vi "Write Data.vi"(8 "error in (no error)":errorcluster, 9 "Publication Time":timestamp, 10 "Value":variant, 11 "FormattedStringBinding In":refnum<class "FormattedStringBinding.lvclass">) -> (0 "error out":errorcluster, 3 "FormattedStringBinding Out":refnum<class "FormattedStringBinding.lvclass">)   [LabVIEW 2019, in "FormattedStringBinding.lvclass"]
doc: "<License>\nCopyright © 2017 Composed Systems, LLC | All rights reserved\nwww.composed.io\n\nAuthor: Ethan Stern <ethan.stern@composed.io>\n\nThis software is provided \"AS IS\" WITHOUT WARRANTIES, either express or implied, AND IS FOR EDUCATIONAL PURPOSES ONLY.\n</License>"
uses:
  <vilib>/gpm_packages/@cs/transport/Source/Concrete/FormattedStringBinding/FormattedStringBinding.lvclass
  <vilib>/gpm_packages/@cs/transport/Source/Concrete/FormattedStringBinding/FormattedStringBinding.lvclass/FormattedStringBinding.ctl
  <vilib>/Utility/error.llb/Error Cluster From Error Code.vi
  <vilib>/gpm_packages/@cs/transport/Source/Concrete/TerminalValueBinding/TerminalValueBinding.lvclass
  <vilib>/ErrorRing/Error Ring.xnode
  <vilib>/Utility/Data Type/NI_Data Type.lvlib
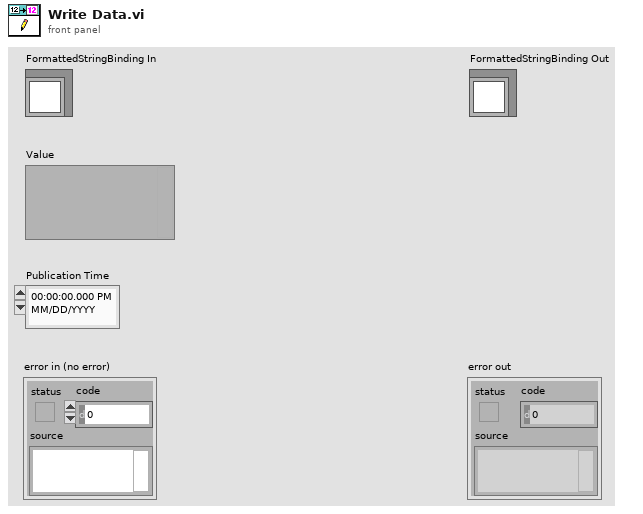
[diagram p1: front panel]
types:
  T1 = typedef "NI_Data Type.lvlib/Data Type.ctl" = enum8{"Invalid Type", "Void", "I8", "I16", "I32", "I64", "U8", "U16", "U32", "U64", "Single Float", "Double Float", "Extended Float", "Single Complex", "Double Complex", "Extended Complex", "Enum U8", "Enum U16", "Enum U32", "Enum U64", "Single Float With Unit", "Double Float With Unit", "Extended Float With Unit", "Single Complex with Unit", "Double Complex with Unit", "Extended Complex with Unit", "Boolean", "String", "Path", "Picture", "Tag", "Array", "Cluster", "Variant", "LV Variant", "Waveform", "Timestamp", "Digital Waveform", "Digital Data", "ExpressData", "Refnum", "External Data", "VI", "Poly VI", "LabVIEW Class Instance", "Fixed Point", "Set Collection", "Map Collection"}
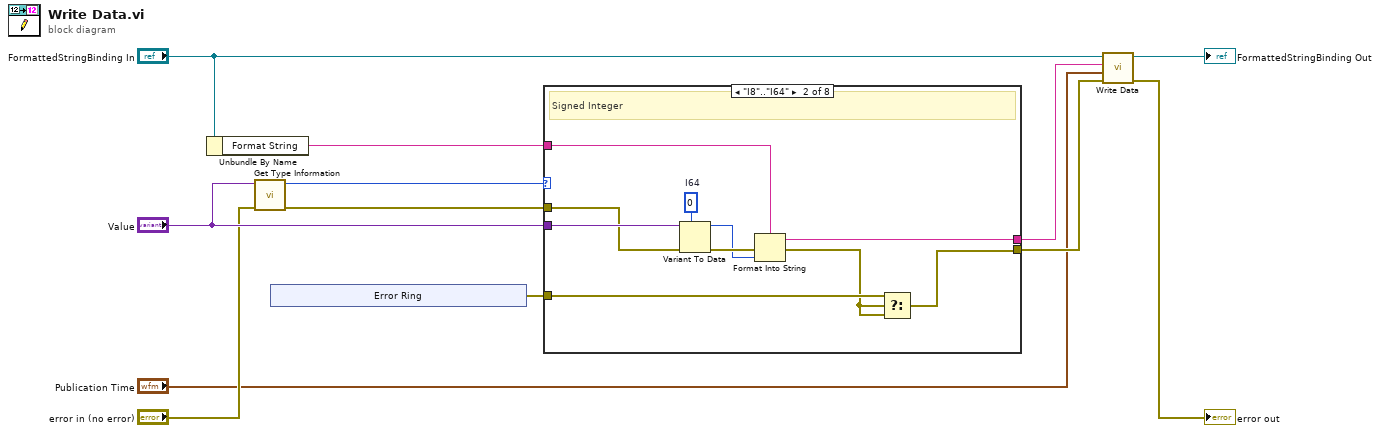
[diagram p0: block diagram]
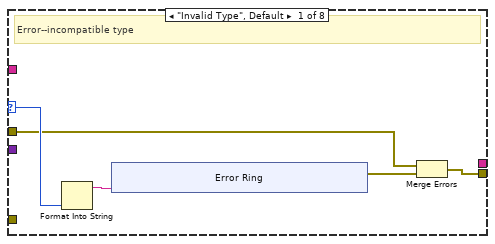
[diagram p2: hidden frame]
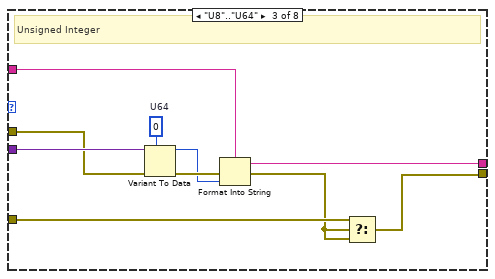
[diagram p3: hidden frame]
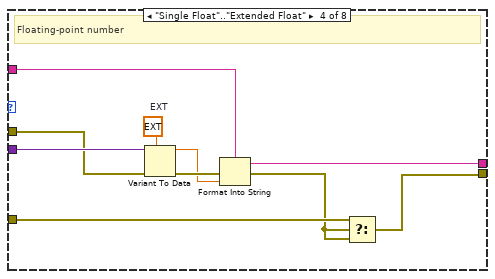
[diagram p4: hidden frame]
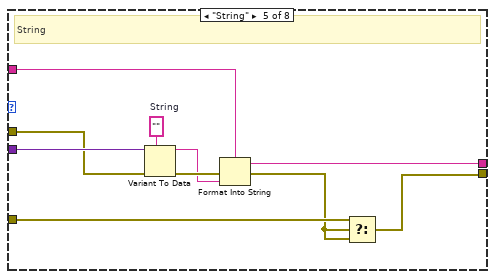
[diagram p5: hidden frame]
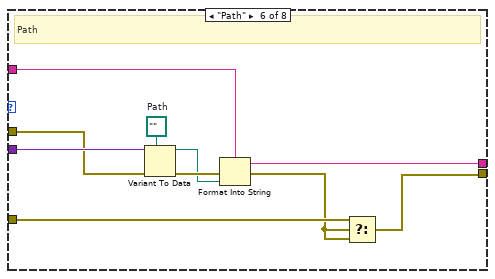
[diagram p6: hidden frame]
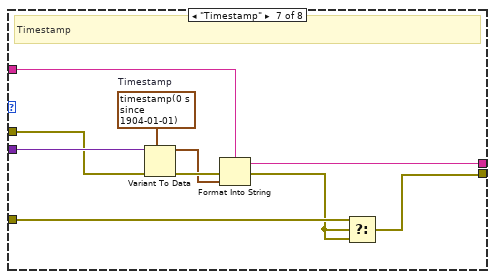
[diagram p7: hidden frame]
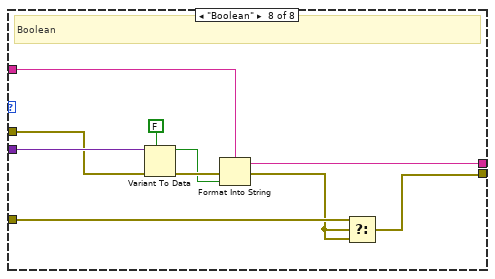
[diagram p8: hidden frame]
diagram:
  n1 = Unbundle By Name("FormattedStringBinding In") -> ("Format String"=w11:string)
  n2 = call <vilib>:"Get Type Information.vi"("error in (no error)"="error in (no error)", "variant"="Value") -> ("error out"=w4:errorcluster, "type"=w9:T1)  [unwired: 5 in, 3 out]
  n3 = xnode "Error Ring"() -> ("error out"=w1:errorcluster)
  n4 = case shown="\"I8\"..\"I64\"" w9 {
    selector: w9 -> [w16 _ _ _ _ _ _ _]
    tunnel: "Value" -> [_ w34 w44 w54 w64 w74 w84 w94]
    tunnel: w11 -> [_ w33 w43 w53 w63 w73 w83 w93]
    tunnel: [w14 w27 w35 w45 w55 w65 w75 w85] -> w7
    tunnel: [_ w31 w41 w51 w61 w71 w81 w91] -> w3
    tunnel: w4 -> [w13 w28 w38 w48 w58 w68 w78 w88]
    tunnel: w1 -> [_ w26 w37 w47 w57 w67 w77 w87]
    frame "Invalid Type", Default {
      # "Error--incompatible type"
      n5 = Format Into String(w16) -> (resulting string=w15:string)  [unwired: 3 in, 1 out]
      n6 = xnode "Error Ring"("parameter 0"=w15) -> ("error out"=w17:errorcluster)
      n7 = Merge Errors(w13, w17) -> (w14:errorcluster)
    }
    frame "I8".."I64" {
      w29 = i64 0  # I64
      # "Signed Integer"
      n8 = Variant To Data(error in=w28, type=w29, Variant=w34) -> (data=w30:i64, error out=w32:errorcluster)
      n9 = Format Into String(format string=w33, error in=w32, w30) -> (resulting string=w31:string, error out=w25:errorcluster)  [unwired: 1 in]
      n10 = Select(t=w26, s=w25, f=w25) -> (s? t:f=w27:errorcluster)
    }
    frame "U8".."U64" {
      w39 = u64 0  # U64
      # "Unsigned Integer"
      n11 = Variant To Data(error in=w38, type=w39, Variant=w44) -> (data=w40:u64, error out=w42:errorcluster)
      n12 = Format Into String(format string=w43, error in=w42, w40) -> (resulting string=w41:string, error out=w36:errorcluster)  [unwired: 1 in]
      n13 = Select(t=w37, s=w36, f=w36) -> (s? t:f=w35:errorcluster)
    }
    frame "Single Float".."Extended Float" {
      w49 = ext 0.0  # EXT
      # "Floating-point number"
      n14 = Variant To Data(error in=w48, type=w49, Variant=w54) -> (data=w50:ext, error out=w52:errorcluster)
      n15 = Format Into String(format string=w53, error in=w52, w50) -> (resulting string=w51:string, error out=w46:errorcluster)  [unwired: 1 in]
      n16 = Select(t=w47, s=w46, f=w46) -> (s? t:f=w45:errorcluster)
    }
    frame "String" {
      w59 = ""  # String
      # "String"
      n17 = Variant To Data(error in=w58, type=w59, Variant=w64) -> (data=w60:string, error out=w62:errorcluster)
      n18 = Format Into String(format string=w63, error in=w62, w60) -> (resulting string=w61:string, error out=w56:errorcluster)  [unwired: 1 in]
      n19 = Select(t=w57, s=w56, f=w56) -> (s? t:f=w55:errorcluster)
    }
    frame "Path" {
      w69 = path ""  # Path
      # "Path"
      n20 = Variant To Data(error in=w68, type=w69, Variant=w74) -> (data=w70:path, error out=w72:errorcluster)
      n21 = Format Into String(format string=w73, error in=w72, w70) -> (resulting string=w71:string, error out=w66:errorcluster)  [unwired: 1 in]
      n22 = Select(t=w67, s=w66, f=w66) -> (s? t:f=w65:errorcluster)
    }
    frame "Timestamp" {
      w79 = timestamp(0 s since 1904-01-01)  # Timestamp
      # "Timestamp"
      n23 = Variant To Data(error in=w78, type=w79, Variant=w84) -> (data=w80:timestamp, error out=w82:errorcluster)
      n24 = Format Into String(format string=w83, error in=w82, w80) -> (resulting string=w81:string, error out=w76:errorcluster)  [unwired: 1 in]
      n25 = Select(t=w77, s=w76, f=w76) -> (s? t:f=w75:errorcluster)
    }
    frame "Boolean" {
      # "Boolean"
      n26 = Variant To Data(error in=w88, type=FALSE, Variant=w94) -> (data=w90:bool, error out=w92:errorcluster)
      n27 = Format Into String(format string=w93, error in=w92, w90) -> (resulting string=w91:string, error out=w86:errorcluster)  [unwired: 1 in]
      n28 = Select(t=w87, s=w86, f=w86) -> (s? t:f=w85:errorcluster)
    }
  }
  n29 = call-parent "Write Data.vi"("error in (no error)"=w7, "Publication Time"="Publication Time", "Value"=w3, "TerminalValueBinding In"="FormattedStringBinding In") -> ("error out"=→"error out":errorcluster, "TerminalValueBinding Out"=→"FormattedStringBinding Out":refnum<class "FormattedStringBinding.lvclass">)  [unwired: 6 in]
